vi "test_fpga_counter.vi"() -> ()   [LabVIEW 2016]
uses:
  <vilib>/Platform/TimedLoop/XDataNode/timing_clust.ctl
  <vilib>/Platform/TimedLoop/XDataNode/nitl_modes.ctl
  <vilib>/Platform/TimedLoop/XDataNode/wakeup.ctl
  <vilib>/Platform/TimedLoop/XDataNode/XDataNode.xnode
  <vilib>/Platform/TimedLoop/XDataNode/XDNodeRunTimeDep.lvlib
panel:
  in  "version2":bool
  in  "doStep":bool=TRUE
  in  "reset":bool
  in  "maxCount":u16
  out "maxReached":bool
  out "maxPulse":bool
  out "next":u16
  out "index":u16
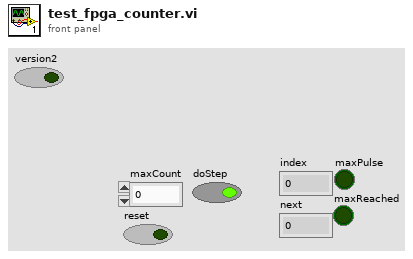
[diagram p1: front panel]
types:
  T1 = typedef "XDNodeRunTimeDep.lvlib/timing_clust.ctl" = cluster{"Expected End [f-1]":u64, "Actual End [f-1]":u64, "Finished Late? [f-1]":bool, "Expected End [i-1]":u64, "Actual End [i-1]":u64, "Finished Late? [i-1]":bool, "Expected Start [i]":u64, "Actual Start [i]":u64, "Expected Start [f]":u64, "Actual Start [f]":u64, "Source Name":string, "Structure Name":string, "Period":i64, "Deadline":i64, "Offset":i64, "Start":i64, "Priority":i32, "Timeout":i32, "Mode":T2, "Wakeup Reason":T3, "Error":errorcluster, "Source Type":string, "Secondary Source Type":string, "Global End Time":u64, "Global Start Time":u64, "Frame Duration":u64, "Iteration Duration":u64, "Assigned CPU":i32, "I/O Scan Engine Mode":u32}
  T2 = typedef "XDNodeRunTimeDep.lvlib/nitl_modes.ctl" = enum32{"No Change", "Process missed periods, maintain original phase", "Discard missed periods, maintain original phase", "Process missed periods, ignore original phase", "Discard missed periods, ignore original phase"}
  T3 = typedef "XDNodeRunTimeDep.lvlib/wakeup.ctl" = enum32{"Normal", "Aborted", "Asynchronous wakeup", "Timing source error", "Timed loop error", "Timeout"}
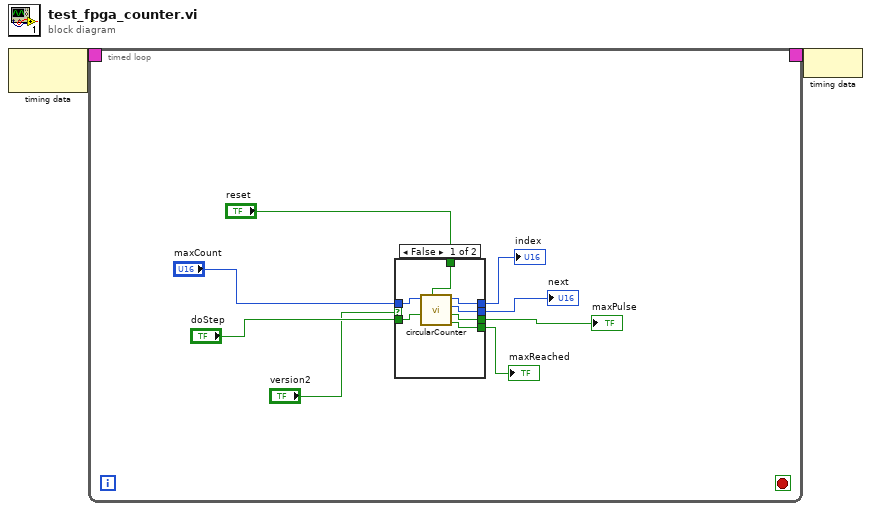
[diagram p0: block diagram]
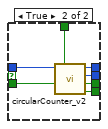
[diagram p2: hidden frame]
diagram:
  n1 = node-c288() -> (w2:T1)  [unwired: 1 in]
  n2 = timed-loop {
    timing: w2 -> [_]
    timing-out: [_] -> w1
    stop <- _ stop-if-true
    n3 = case shown="False" "version2" {
      tunnel: "maxCount" -> [w17 w24]
      tunnel: "doStep" -> [w16 w23]
      tunnel: "reset" -> [w15 w22]
      tunnel: [w14 w21] -> w7
      tunnel: [w13 w20] -> w6
      tunnel: [w12 w19] -> w5
      tunnel: [w11 w18] -> w4
      frame False {
        n4 = call "circularCounter.vi"("reset"=w15, "doStep"=w16, "maxCount"=w17) -> ("maxReached"=w11:bool, "maxPulse"=w12:bool, "next"=w13:u16, "index"=w14:u16)  [unwired: 5 in]
      }
      frame True {
        n5 = call "circularCounter_v2.vi"("reset"=w22, "doStep"=w23, "maxCount"=w24) -> ("maxReached"=w18:bool, "maxPulse"=w19:bool, "next"=w20:u16, "index"=w21:u16)  [unwired: 5 in]
      }
    }
    "index" <- w7
    "next" <- w6
    "maxPulse" <- w5
    "maxReached" <- w4
  }
  n6 = node-c288(w1) -> ()
